vi "Initialize Device.vi"(8 "Error In":errorcluster, 9 "TCP Configuration":T3, 10 "COM Port":refnum<visa-resource-name>, 11 "Interface":T2) -> (0 "Error Out":errorcluster, 3 "LINX Device Config":T1)   [LabVIEW 2011, in "LVH-LINX.lvlib"]
uses:
  LVH-LINX.lvlib
  Private/Type Defs/TCP Config.ctl
  Private/Type Defs/Interface.ctl
  Private/Type Defs/LINX Device Config.ctl
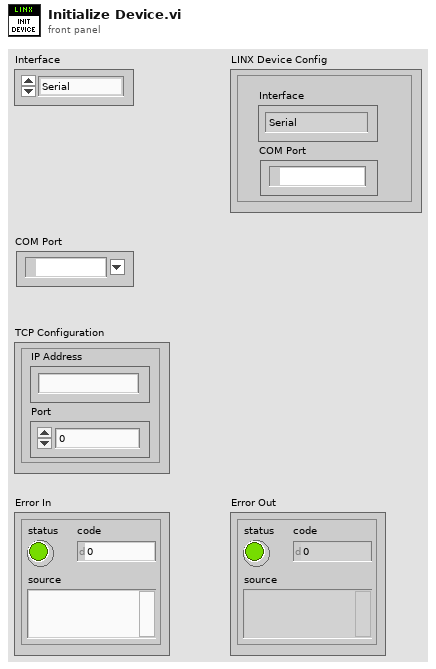
[diagram p1: front panel]
types:
  T1 = typedef "LVH-LINX.lvlib/LINX Device Config.ctl" = cluster{"Interface":T2, "COM Port":refnum<visa-resource-name>, "Packet Number":u16, "TCP Configuration":T3}
  T2 = typedef "LVH-LINX.lvlib/Interface.ctl" = enum16{"Serial", "TCP"}
  T3 = typedef "LVH-LINX.lvlib/TCP Config.ctl" = cluster{"IP Address":string, "Port":dbl}
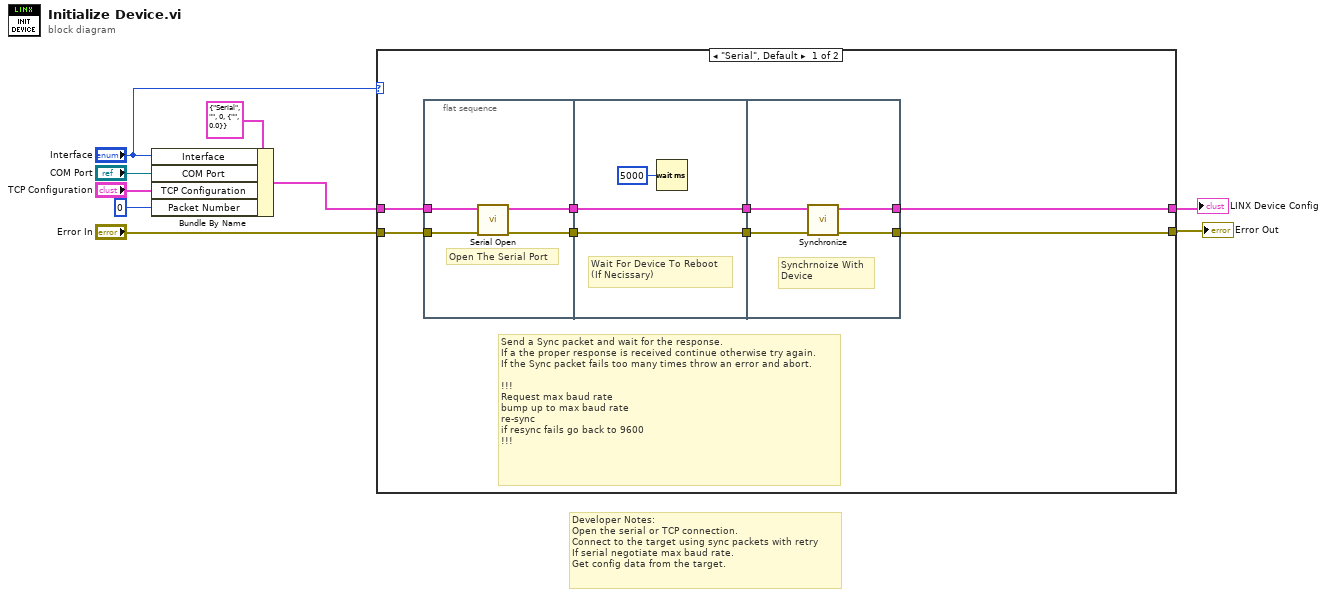
[diagram p0: block diagram]
diagram:
  # "Developer Notes:\nOpen the serial or TCP connection.\nConnect to the target using sync packets with retry\nIf serial negotiate max baud rate.\nGet config data from the target."
  n1 = Bundle By Name(cluster=T1 {"Interface"=enum."Serial", "COM Port"="", "Packet Number"=0, "TCP Configuration"={"IP Address"="", "Port"=0.0}} ("LINX Device Config"), "Interface"="Interface", "COM Port"="COM Port", "TCP Configuration"="TCP Configuration", "Packet Number"=u16 0) -> (w4:T1)
  n2 = case shown="\"Serial\", Default" "Interface" {
    tunnel: "Error In" -> [w17 w30]
    tunnel: [w10 w30] -> w1
    tunnel: w4 -> [w16 w29]
    tunnel: [w11 w29] -> w2
    frame "Serial", Default {
      # "Send a Sync packet and wait for the response.\nIf a the proper response is received continue otherwise try again.\nIf the Sync packet fails too many times throw an error and abort.\n\n!!!\nRequest max baud rate\nbump up to max baud rate\nre-sync\nif resync fails go back to 9600\n!!!"
      n3 = flat-sequence {
        tunnel: w17 -> [w21]
        tunnel: w16 -> [w20]
        tunnel: [w19] -> w15
        tunnel: [w18] -> w12
        tunnel: w15 -> [w23]
        tunnel: [w23] -> w14
        tunnel: [w22] -> w13
        tunnel: w12 -> [w22]
        tunnel: w14 -> [w28]
        tunnel: w13 -> [w27]
        tunnel: [w26] -> w11
        tunnel: [w25] -> w10
        frame #0 {
          # "Open The Serial Port"
          n4 = call "Serial Open.vi"("Error In"=w21, "LINX Device Config"=w20) -> ("Error Out"=w18:errorcluster, "LINX Device Config"=w19:T1)  [unwired: 8 in]
        }
        frame #1 {
          # "Wait For Device To Reboot\n(If Necissary)"
          n5 = Wait (ms)(milliseconds to wait=u32 5000) -> ()  [unwired: 1 out]
        }
        frame #2 {
          # "Synchrnoize With\nDevice"
          n6 = call "Synchronize.vi"("Error In"=w27, "LINX Device Config"=w28) -> ("Error Out"=w25:errorcluster, "LINX Device Config"=w26:T1)  [unwired: 8 in]
        }
      }
    }
    frame "TCP" {
      # "Add TCP Case Here!!!"
    }
  }
  "Error Out" <- w1
  "LINX Device Config" <- w2
